vi "Generate a Pulse.vi"() -> ()   [LabVIEW 2021]
panel:
  in  "stop":bool
  in  "device name":tag="Dev1"
  in  "Sample":bool
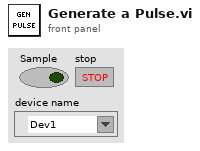
[diagram p1: front panel]
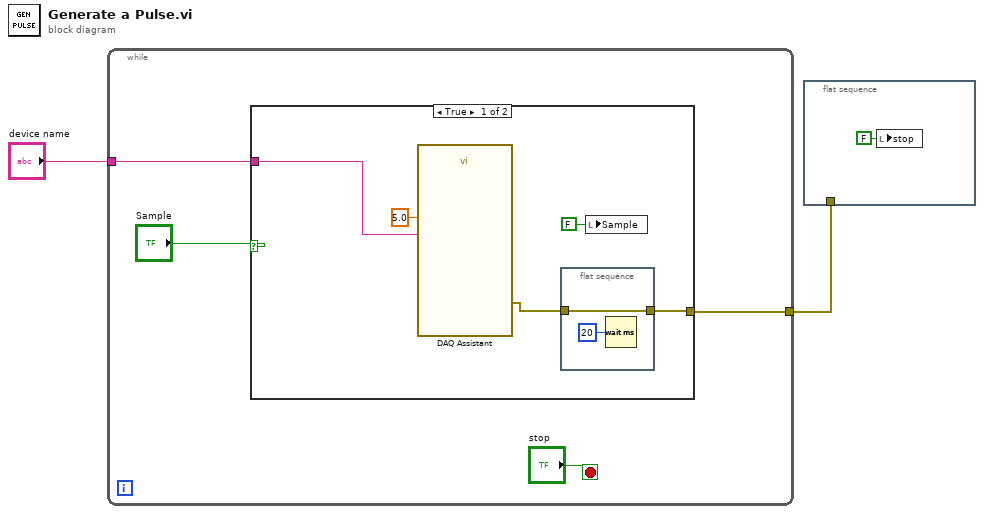
[diagram p0: block diagram]
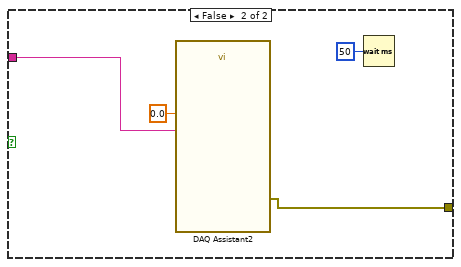
[diagram p2: hidden frame]
diagram:
  n1 = while {
    tunnel: "device name" -> [w5]
    tunnel: [w3] -> w1
    stop <- "stop" stop-if-true
    n2 = case shown="True" "Sample" {
      tunnel: w5 -> [w11 w17]
      tunnel: [w8 w15] -> w3
      frame True {
        n3 = call "DAQ Assistant"("data"=5.0, "device name"=w11) -> ("error out"=w7:errorcluster)  [unwired: 16 in, 1 out]
        n4 = flat-sequence {
          tunnel: [w13] -> w8
          tunnel: w7 -> [w13]
          frame #0 {
            n5 = Wait (ms)(milliseconds to wait=u32 20) -> ()  [unwired: 1 out]
          }
        }
        n6 = local write "Sample"(FALSE ("Sample")) -> ()
      }
      frame False {
        n7 = call "DAQ Assistant2"("data"=0.0, "device name"=w17) -> ("error out"=w15:errorcluster)  [unwired: 16 in, 1 out]
        n8 = Wait (ms)(milliseconds to wait=u32 50) -> ()  [unwired: 1 out]
      }
    }
  }
  n9 = flat-sequence {
    tunnel: w1 -> [_]
    frame #0 {
      n10 = local write "stop"(FALSE ("stop")) -> ()
    }
  }
